vi "finish.vi"(11 "ActiveSuspension.lvclass":refnum<class "System.lvclass">) -> (0 "error out":errorcluster)   [LabVIEW 2021, in "System.lvclass"]
uses:
  System.lvclass
  System.lvclass/System.ctl
  <vilib>/myRIO/Common/Instrument Driver Framework/myRIO v1.0/UART/vis/myRIO v1.0 Close UART.vi
  <vilib>/myRIO/Common/Instrument Driver Framework/Utilities/vis/FPGA Ref Manager.vi
  <vilib>/myRIO/Common/Instrument Driver Framework/myRIO v1.0/myRIO v1.0 Reset FPGA.vi
  <vilib>/myRIO/Common/Instrument Driver Framework/myRIO v1.0/IRQ/vis/myRIO v1.0 IRQ Info FGV.vi
  <vilib>/myRIO/Common/Instrument Driver Framework/myRIO v1.0/IRQ/vis/myRIO v1.0 Timer IRQ Info FGV.vi
  <vilib>/myRIO/Common/Instrument Driver Framework/myRIO v1.0/IRQ/vis/myRIO v1.0 ISR Agent.vi
  <vilib>/myRIO/Instrument Drivers/Utilities/vis/Reset Index.vi
  <vilib>/myRIO/Common/Instrument Driver Framework/myRIO v1.0/Resource Manager/vis/myRIO v1.0 Block Write Resource Manager.vi
  <vilib>/myRIO/Instrument Drivers/Utilities/Utilities.lvlib
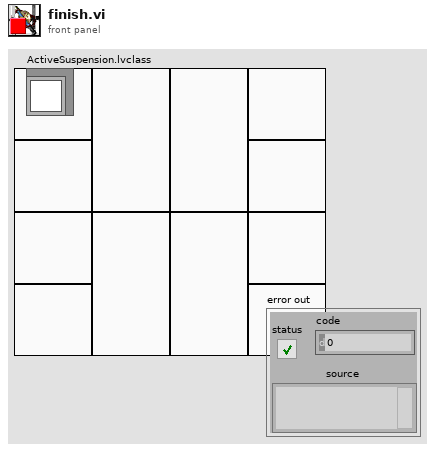
[diagram p1: front panel]
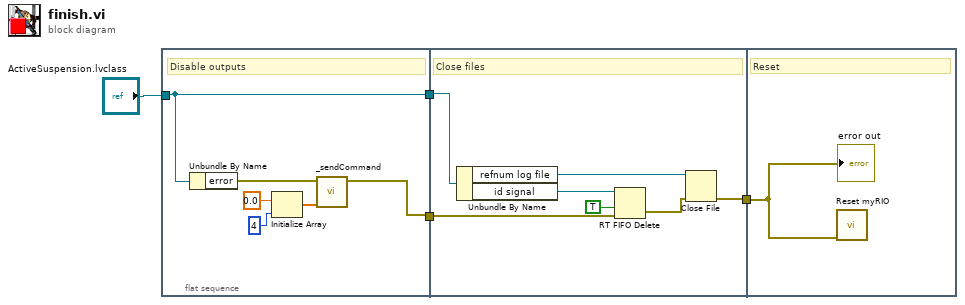
[diagram p0: block diagram]
diagram:
  n1 = flat-sequence {
    tunnel: "ActiveSuspension.lvclass" -> [w5]
    tunnel: [w5] -> w3
    tunnel: [w6] -> w2
    tunnel: w3 -> [w14]
    tunnel: w2 -> [w13]
    tunnel: [w12] -> w1
    tunnel: w1 -> [w18]
    frame #0 {
      # "Disable outputs"
      n2 = Unbundle By Name(w5) -> ("error"=w10:errorcluster)
      n3 = Initialize Array(0.0 ("element"), 4 ("dimension size")) -> (w7:dbl[])
      n4 = call "_sendCommand.vi"("FBLR"=w7, "error in (no error)"=w10) -> ("error out"=w6:errorcluster)  [unwired: 9 in]
    }
    frame #1 {
      # "Close files"
      n5 = Unbundle By Name(w14) -> ("refnum log file"=w17:refnum<file>, "id signal"=w16:refnum<k33>)
      n6 = RT FIFO Delete(0:w16, 2:TRUE ("force destroy? (F)"), 3:w13) -> (11:w15:errorcluster)
      n7 = Close File(refnum=w17, error in=w15) -> (error out=w12:errorcluster)  [unwired: 1 out]
    }
    frame #2 {
      # "Reset"
      n8 = call <vilib>:"Reset myRIO.vi"("error in (no error)"=w18) -> ()  [unwired: 10 in, 1 out]
      "error out" <- w18
    }
  }
